vi "Set and Get Disp.vi"(7 "Mode":T2, 8 "错误输入":errorcluster, 10 "显示项输入":T1={"垂直滚动条"=FALSE, "水平滚动条"=FALSE, "行首"=TRUE, "列首"=FALSE, "垂直线"=FALSE, "水平线"=TRUE, "符号"=TRUE}, 11 "Mlistbox Ref":refnum<vi>) -> (0 "错误输出":errorcluster, 2 "显示项输出":T1={"垂直滚动条"=FALSE, "水平滚动条"=FALSE, "行首"=TRUE, "列首"=FALSE, "垂直线"=FALSE, "水平线"=TRUE, "符号"=TRUE}, 3 "Mlistbox Ref Dup":refnum<vi>)   [LabVIEW 2012, in "Mlistbox Tools.lvlib"]
uses:
  Mlistbox Tools.lvlib
  ListBox/Custom Type/Read and Write Mode.ctl
  Custom Type/Disp.ctl
  ListBox/Listbox Tool.lvlib
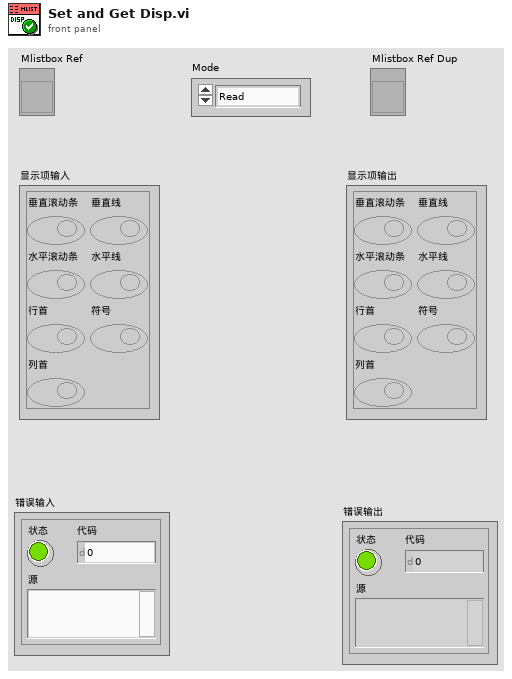
[diagram p1: front panel]
types:
  T1 = typedef "Mlistbox Tools.lvlib/Disp.ctl" = cluster{"垂直滚动条":bool, "水平滚动条":bool, "行首":bool, "列首":bool, "垂直线":bool, "水平线":bool, "符号":bool}
  T2 = typedef "Listbox Tool.lvlib/Read and Write Mode.ctl" = enum16{"Read", "Write"}
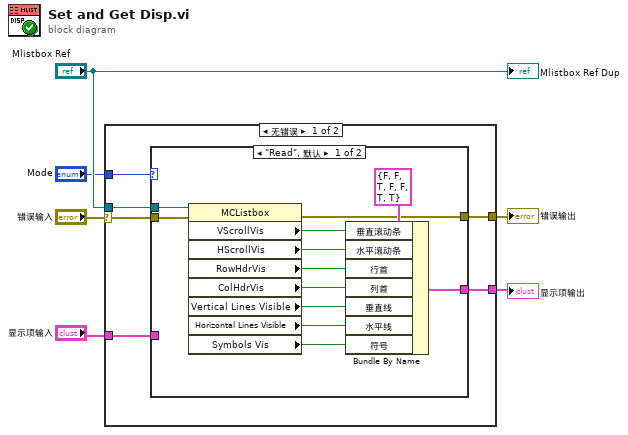
[diagram p0: block diagram]
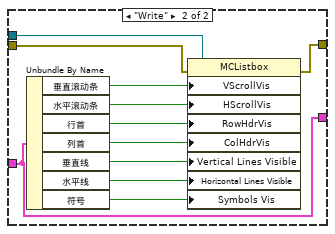
[diagram p2: hidden frame]
diagram:
  n1 = case shown="无错误" "错误输入" {
    selector: "错误输入" -> [w10 w36]
    tunnel: [w9 w36] -> w5
    tunnel: "Mlistbox Ref" -> [w11 _]
    tunnel: "Mode" -> [w12 _]
    tunnel: "显示项输入" -> [w8 _]
    tunnel: [w7 _] -> w1
    frame No Error {
      n2 = case shown="\"Read\", 默认" w12 {
        tunnel: w11 -> [w23 w35]
        tunnel: w10 -> [w24 w34]
        tunnel: [w20 w33] -> w9
        tunnel: w8 -> [_ w25]
        tunnel: [w21 w25] -> w7
        frame "Read", Default {
          n3 = property class="MCListbox"(reference=w23, error in=w24) -> (error out=w20:errorcluster, "VScrollVis"=w19:bool, "HScrollVis"=w18:bool, "RowHdrVis"=w17:bool, "ColHdrVis"=w16:bool, "Vertical Lines Visible"=w15:bool, "Horizontal Lines Visible"=w14:bool, "Symbols Vis"=w13:bool)  [unwired: 1 out]
          n4 = Bundle By Name(cluster=T1 {"垂直滚动条"=FALSE, "水平滚动条"=FALSE, "行首"=TRUE, "列首"=FALSE, "垂直线"=FALSE, "水平线"=TRUE, "符号"=TRUE} ("显示项输入"), "垂直滚动条"=w19, "水平滚动条"=w18, "行首"=w17, "列首"=w16, "垂直线"=w15, "水平线"=w14, "符号"=w13) -> (w21:T1)
        }
        frame "Write" {
          n5 = Unbundle By Name(w25) -> ("垂直滚动条"=w32:bool, "水平滚动条"=w31:bool, "行首"=w30:bool, "列首"=w29:bool, "垂直线"=w28:bool, "水平线"=w27:bool, "符号"=w26:bool)
          n6 = property class="MCListbox"(reference=w35, error in=w34, "VScrollVis"=w32, "HScrollVis"=w31, "RowHdrVis"=w30, "ColHdrVis"=w29, "Vertical Lines Visible"=w28, "Horizontal Lines Visible"=w27, "Symbols Vis"=w26) -> (error out=w33:errorcluster)  [unwired: 1 out]
        }
      }
    }
    frame Error {
    }
  }
  "错误输出" <- w5
  "显示项输出" <- w1
  "Mlistbox Ref Dup" <- "Mlistbox Ref"
